vi "Fuel Refinement.vi"() -> ()   [LabVIEW 2023]
panel:
  in  "Chem. Dissolution Gas":u32 max=8
  out "UF6 Limiting":bool
  in  "Centrifuge Speed":u32 max=8
  out "UF6 (mB/t)":ext format="%.2f"
  out "Self Limiting":bool
  out "UO Limiting":bool
  out "HF Limiting":bool
  out "HF (mB/t)":ext format="%.2f"
  out "UO (mB/t)":ext format="%.2f"
  out "UF6 (mB/t)":ext format="%.2f"
  in  "Chem. Infuser Speed":u32 max=8
  out "Fluorite/s":ext
  out "Uranium Ingots/s":ext
  out "Yellow Cake/t":ext
  in  "Enrichment Speed":u32 max=8
  out "YK Limiting":bool
  out "Self Limiting":bool
  out "UO2 (mB/t)":ext format="%.2f"
  in  "Ox Speed":u32 max=8
  out "Coal/s":ext
  out "HF (mB/t)":u32
  out "H2SO4 Limiting":bool
  out "Self Limiting":bool
  out "H2SO4 (mB/t)":ext format="%.2f"
  in  "Chem. Dissolution Speed":u32 max=8
  out "Fluorite/t":ext
  out "Self Limiting":bool
  out "H2O Limiting":bool
  out "SO3 Limiting":bool
  out "SO3 (mB/t)":ext format="%.2f"
  out "H2O Vapor (mB/t)":ext format="%.2f"
  out "Sulfur Dust/t":ext
  out "H2SO4 (mB/t)":ext format="%.2f"
  in  "Chem. Infuser Speed":u32 max=8
  out "H2O Vapor (mB/t)":u32
  in  "Rotary Cond. Speed":u32 max=8
  out "SO3 (mB/t)":ext format="%.2f"
  out "Self Limiting":bool
  out "SO2 Limiting":bool
  out "O Limiting":bool
  out "O (mB/t)":ext format="%.2f"
  out "SO2 (mB/t)":ext format="%.2f"
  in  "Chem. Infuser Speed":u32 max=8
  out "H (mB/t)":u32
  out "O (mB/t)":u32
  in  "E.S. Speed":u32 max=8
  out "Dust Limiting":bool
  out "Self Limiting":bool
  out "SO2 (mB/t)":ext format="%.2f"
  in  "Ox Speed":u32 max=8
  out "H (mB/t)":u32
  out "O (mB/t)":u32
  out "Self Limiting":bool
  out "PRC O Limiting":bool
  out "PRC H2O Limiting":bool
  in  "P.R.C. Speed":u32 max=8
  in  "E.S. Speed":u32 max=8
  out "Coal/t":ext
  out "Self Limiting":bool
  out "Fissile Fuel (mB/t)":ext
  out "Uranium Ingots/t":ext
  # "Input Requirements"
  # "Sulfur Elec. Separator"
  # "Sulfur Elec. Separator"
  # "Water Vapor"
  # "Input Requirements"
  # "Sulfur Production"
  # "Sulfur Dioxide"
  # "Sulfur Trixoide"
  # "Sulfuric Acid"
  # "Yellow Cake Production"
  # "Uranium Oxide"
  # "Uranium Hexafluoride"
  # "Hydrofluoric Acid"
  # "Fissile Fuel"
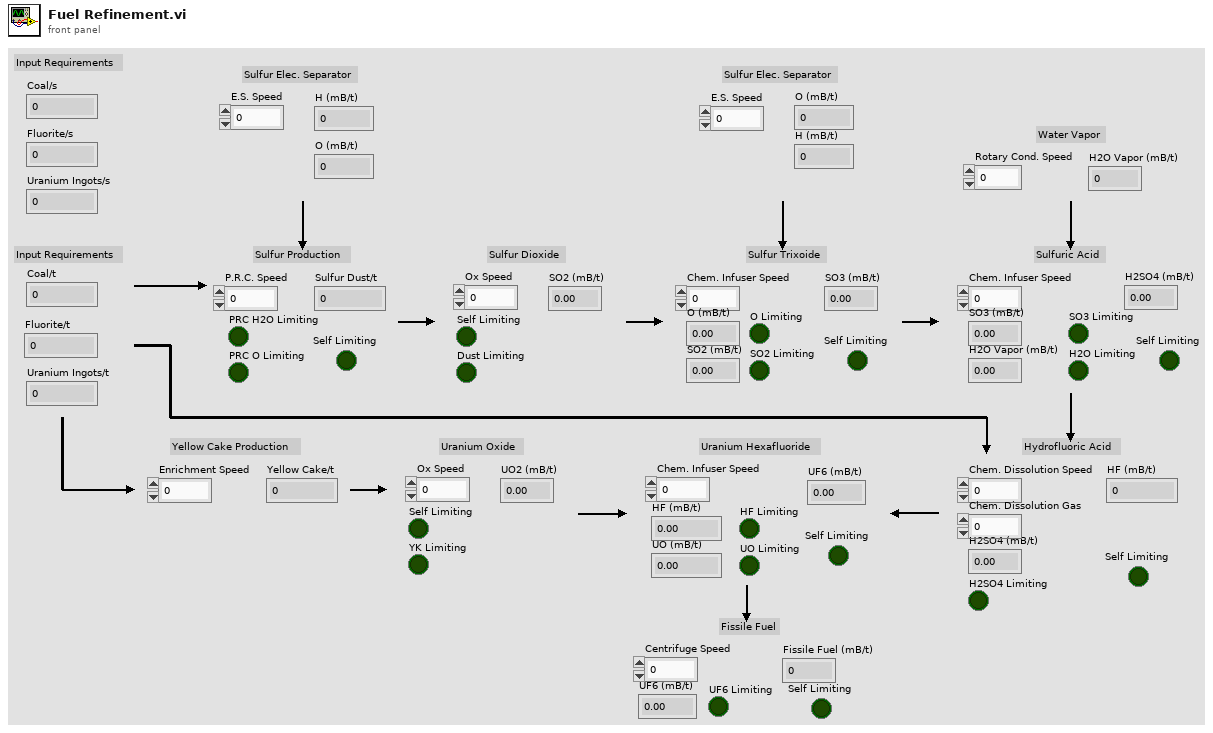
[diagram p1: front panel]
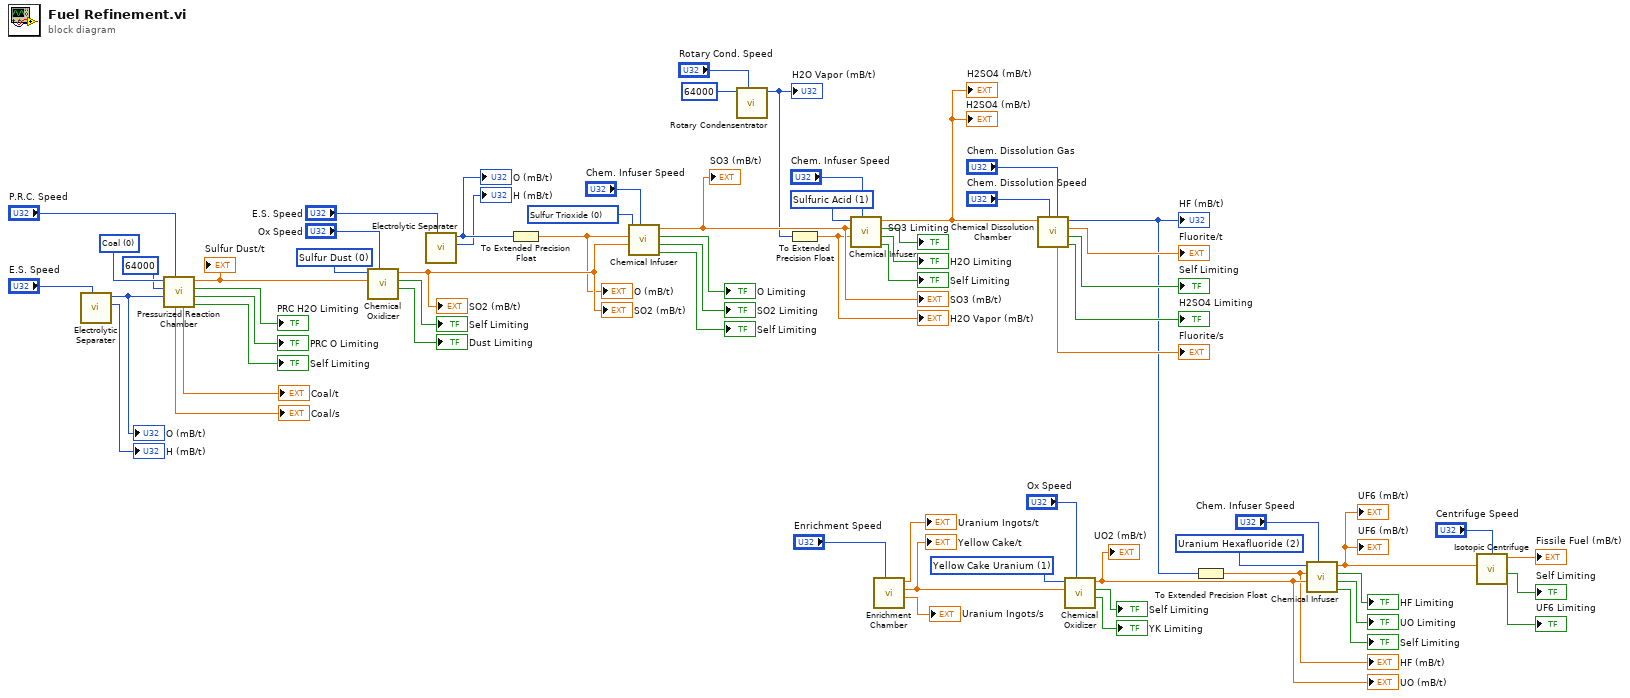
[diagram p0: block diagram]
diagram:
  w52 = u16 0 items=["Sulfur Trioxide", "Sulfuric Acid", "Uranium Hexafluoride"] ("Recipe")
  w56 = u16 0 items=["Sulfur Dust", "Yellow Cake Uranium", "Yellow Cake Uranium Block"] ("Input")
  w59 = u16 1 items=["Sulfur Trioxide", "Sulfuric Acid", "Uranium Hexafluoride"] ("Recipe")
  w61 = u16 2 items=["Sulfur Trioxide", "Sulfuric Acid", "Uranium Hexafluoride"] ("Recipe")
  w63 = u16 0 items=["Coal", "Coal Block"] ("Input")
  w64 = u16 1 items=["Sulfur Dust", "Yellow Cake Uranium", "Yellow Cake Uranium Block"] ("Input")
  n1 = call "Electrolytic Separater.vi"("Speed Upgrades"="E.S. Speed") -> ("Hydrogen (mB/t)"=→"H (mB/t)":u32, "Oxygen (mB/t)"=w54:u32)  [unwired: 6 in]
  "O (mB/t)" <- w54
  n2 = call "Pressurized Reaction Chamber.vi"("Speed Upgrades"="P.R.C. Speed", "In Gas (mB/t)"=w54, "Water (mB/t)"=u32 64000, "Input"=w63) -> ("Limiting"=→"Self Limiting":bool, "B Limiting"=→"PRC O Limiting":bool, "A Limiting"=→"PRC H2O Limiting":bool, "Produced Items/t"=w55:ext, "Required Items/t"=→"Coal/t":ext, "Required Items/s"=→"Coal/s":ext)  [unwired: 1 in, 1 out]
  "Sulfur Dust/t" <- w55
  n3 = call "Chemical Oxidizer.vi"("Speed Upgrades"="Ox Speed", "Items/t In"=w55, "Input"=w56) -> ("Input Limiting"=→"Dust Limiting":bool, "Limiting"=→"Self Limiting":bool, "Output Gas (mB/t)"=w4:ext)  [unwired: 4 in, 2 out]
  "SO2 (mB/t)" <- w4
  "SO2 (mB/t)" <- w4
  n4 = call "Electrolytic Separater.vi"("Speed Upgrades"="E.S. Speed") -> ("Hydrogen (mB/t)"=→"H (mB/t)":u32, "Oxygen (mB/t)"=w51:u32)  [unwired: 6 in]
  "O (mB/t)" <- w51
  n5 = To Extended Precision Float(1:w51) -> (0:w3:ext)
  "O (mB/t)" <- w3
  n6 = call "Chemical Infuser.vi"("Speed Upgrades"="Chem. Infuser Speed", "Gas B (mB/t)"=w4, "Gas A (mB/t)"=w3, "Recipe"=w52) -> ("Limiting"=→"Self Limiting":bool, "B Limiting"=→"SO2 Limiting":bool, "A Limiting"=→"O Limiting":bool, "Output Gas (mB/t)"=w28:ext)  [unwired: 4 in]
  "SO3 (mB/t)" <- w28
  "SO3 (mB/t)" <- w28
  n7 = call "Rotary Condensentrator.vi"("Speed Upgrades"="Rotary Cond. Speed", "Liquid (mB/t)"=u32 64000) -> ("Gas (mB/t)"=w27:u32)  [unwired: 8 in, 1 out]
  "H2O Vapor (mB/t)" <- w27
  n8 = To Extended Precision Float(1:w27) -> (0:w2:ext)
  "H2O Vapor (mB/t)" <- w2
  n9 = call "Chemical Infuser.vi"("Speed Upgrades"="Chem. Infuser Speed", "Gas B (mB/t)"=w2, "Gas A (mB/t)"=w28, "Recipe"=w59) -> ("Limiting"=→"Self Limiting":bool, "B Limiting"=→"H2O Limiting":bool, "A Limiting"=→"SO3 Limiting":bool, "Output Gas (mB/t)"=w1:ext)  [unwired: 4 in]
  "H2SO4 (mB/t)" <- w1
  "H2SO4 (mB/t)" <- w1
  n10 = call "Enrichment Chamber.vi"("Speed Upgrades"="Enrichment Speed") -> ("Uranium Ingots/s"=→"Uranium Ingots/s":ext, "Yellow Cake/t"=w60:ext, "Uranium Ingots/t"=→"Uranium Ingots/t":ext)  [unwired: 7 in, 1 out]
  "Yellow Cake/t" <- w60
  n11 = call "Chemical Dissolution Chamber.vi"("Gas Upgrades"="Chem. Dissolution Gas", "Speed Upgrades"="Chem. Dissolution Speed", "Sulfuric Acid (mB/t)"=w1) -> ("Input Limiting"=→"H2SO4 Limiting":bool, "Limiting"=→"Self Limiting":bool, "Required Items/t"=→"Fluorite/t":ext, "Hydrofluoric Acid (mB/t)"=w13:u32, "Required Items/s"=→"Fluorite/s":ext)  [unwired: 3 in, 1 out]
  "HF (mB/t)" <- w13
  n12 = call "Chemical Oxidizer.vi"("Speed Upgrades"="Ox Speed", "Items/t In"=w60, "Input"=w64) -> ("Input Limiting"=→"YK Limiting":bool, "Limiting"=→"Self Limiting":bool, "Output Gas (mB/t)"=w6:ext)  [unwired: 4 in, 2 out]
  "UO2 (mB/t)" <- w6
  "UO (mB/t)" <- w6
  n13 = To Extended Precision Float(1:w13) -> (0:w5:ext)
  "HF (mB/t)" <- w5
  n14 = call "Chemical Infuser.vi"("Speed Upgrades"="Chem. Infuser Speed", "Gas B (mB/t)"=w6, "Gas A (mB/t)"=w5, "Recipe"=w61) -> ("Limiting"=→"Self Limiting":bool, "B Limiting"=→"UO Limiting":bool, "A Limiting"=→"HF Limiting":bool, "Output Gas (mB/t)"=w10:ext)  [unwired: 4 in]
  "UF6 (mB/t)" <- w10
  "UF6 (mB/t)" <- w10
  n15 = call "Isotopic Centrifuge.vi"("Speed Upgrades"="Centrifuge Speed", "Uranium Hexaflouride (mB/t)"=w10) -> ("Input Limiting"=→"UF6 Limiting":bool, "Limiting"=→"Self Limiting":bool, "Fissile Fuel (mB/t)"=→"Fissile Fuel (mB/t)":ext)  [unwired: 4 in]
